vi "Launch Target Actor.vi"() -> ()   [LabVIEW 2023]
uses:
  CRIO MSS Test Actor/CRIO MSS Test Actor.lvclass
  CRIO MSS Test Actor/CRIO MSS Test Actor.lvclass/CRIO MSS Test Actor.ctl
  <vilib>/ni/Actors/Network Endpoint Actors/Protocols/Network Stream Strategy/Netowrk Stream Listener/Network Stream Listener.lvclass
  <vilib>/ActorFramework/Actor/Actor.lvclass
  DIO/DO DAQmx Fixed Freq PWM CFG/DO DAQmx Fixed Freq PWM CFG.lvclass
  Thermometer/Thermometer DAQmx Base CFG/Thermometer DAQmx Base CFG.lvclass
panel:
  out "error out":errorcluster
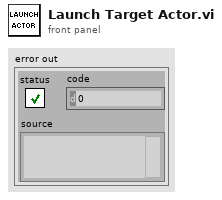
[diagram p1: front panel]
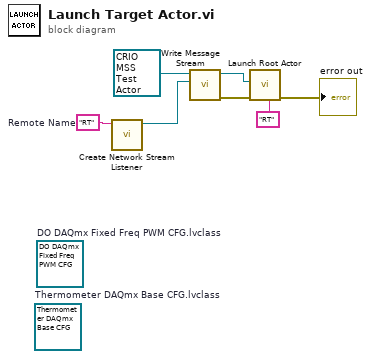
[diagram p0: block diagram]
diagram:
  (unwired) refnum<class "Thermometer DAQmx Base CFG.lvclass"> refnum  # Thermometer DAQmx Base CFG.lvclass
  (unwired) refnum<class "DO DAQmx Fixed Freq PWM CFG.lvclass"> refnum  # DO DAQmx Fixed Freq PWM CFG.lvclass
  w7 = "RT"  # Remote Name
  n1 = call <vilib>:"Create Network Stream Listener.vi"("Name"=w7) -> ("Network Stream Listener"=w5:refnum<class "Network Stream Listener.lvclass">)  [unwired: 10 in]
  n2 = call "Write Message Stream.vi"("Message Stream.lvclass"=w5, "CRIO MSS Test Actor in"=refnum<class "CRIO MSS Test Actor.lvclass"> refnum ("CRIO MSS Test Actor.lvlib:CRIO MSS Test Actor.lvclass")) -> ("error out"=w4:errorcluster, "CRIO MSS Test Actor out"=w3:refnum<class "CRIO MSS Test Actor.lvclass">)  [unwired: 8 in]
  n3 = call <vilib>:"Launch Root Actor.vi"("Debug Alias"="RT", "error in (no error)"=w4, "Actor"=w3) -> ("error out"=→"error out":errorcluster)  [unwired: 7 in, 1 out]
